vi "Handle Error.vi"(8 "error in (no error)":errorcluster, 11 "MSS Host Actor in":refnum<class "MSS Host Actor.lvclass">) -> (0 "error out":errorcluster, 2 "stop actor?":bool=TRUE, 3 "MSS Host Actor out":refnum<class "MSS Host Actor.lvclass">)   [LabVIEW 2023, in "MSS Host Actor.lvlib" / "MSS Host Actor.lvclass"]
doc: "(<B>Filename</B>: Actor Framework.lvlib:Actor.lvclass:Handle Error.vi)\n\nDefines how the actor handles an error that occurred while processing a message. By default, this method does nothing except stop the actor."
uses:
  MSS Host Actor.lvclass
  MSS Host Actor.lvclass/MSS Host Actor.ctl
  <vilib>/ActorFramework/Actor/Actor.lvclass
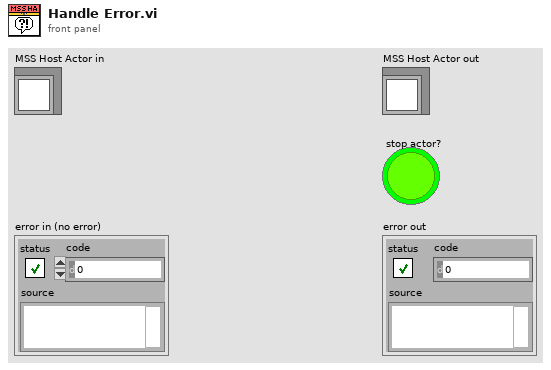
[diagram p1: front panel]
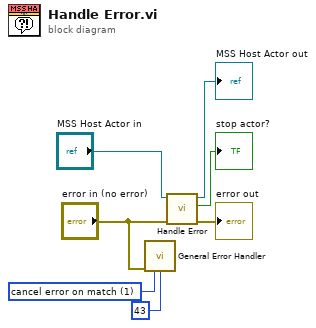
[diagram p0: block diagram]
diagram:
  w2 = 1 items=["no exception", "cancel error on match", "set error on match"] ("[exception action] (none:0)")
  n1 = call <vilib>:"General Error Handler.vi"("error in (no error)"="error in (no error)", "[exception action] (none:0)"=w2, "[exception code]"=43) -> ()  [unwired: 8 in, 5 out]
  n2 = call-parent "Handle Error.vi"("error in (no error)"="error in (no error)", "Actor in"="MSS Host Actor in") -> ("error out"=→"error out":errorcluster, "stop actor?"=→"stop actor?":bool, "Actor out"=→"MSS Host Actor out":refnum<class "MSS Host Actor.lvclass">)  [unwired: 7 in]
